vi "Write Read Loop with Config Speed Test eNames.vi"() -> (0 "error out":errorcluster)   [LabVIEW 2020]
panel:
  out "aValuesOut":dbl[][](array[numeric]) format="%.2f"
  in  "aNumValues":i32[](array[numeric])=[1, 1, 1, 1]
  in  "aWrites":i32[](array[ring])=[1, 1, 0, 0] items=["Read", "Write"]
  in  "aValuesIn":dbl[][](array[numeric])=[[2.34], [1.0]] format="%.2f"
  in  "aNames":string[](array[string])=["DAC0", "FIO1", "AIN0", "AIN1"]
  out "min ms":ext format="%.3g"
  out "max ms":ext format="%.3g"
  out "avg ms per iteration":ext format="%.3f"
  out "total ms":ext format="%.3g"
  out "Interval Array [ms] (Sorted Descending)":ext[](array[numeric]) format="%.3g"
  in  "Enable Interval Timing":bool=TRUE
  out "Interval Array [ms]":ext[](array[numeric]) format="%.3g"
  in  "# Iterations":i32=1000
  in  "Config Values":dbl[](array[numeric])=[10.0, 1.0] format="%.2f"
  in  "Config Names":string[](array[string])=["AIN_ALL_RANGE", "AIN_ALL_RESOLUTION_INDEX"]
  in  "Interval [ms]":i32
  out "Error String":string
  out "ConnectionType Out":i32
  out "DeviceType Out":i32
  in  "Identifier":string="LJM_idANY"
  in  "ConnectionType":string="LJM_ctANY"
  in  "DeviceType":string="LJM_dtANY"
  # "This modified version of a basic example adds code to do interval timing.  It does\nthe specified number of iterations and reports the average time per iteration.\n\nSet controls as desired then click arrow (upper-left of window) to run.  First the device is set to factory condition.  Then config values are written once before the loop.  Set Interval=0 to run as fast as possible.\n\nThis version uses 1 call to eNames to write and read."
  # "To remove an element, right-click on it, select\nData Operations => Remove Element.\n\nTo empty an array, right-click near the edge, select\nData Operations => Empty Array.\n\nOther useful operations:  From the Operate menu are \"Make Current\nValues Default\" and \"Reinitialize To Default\" (source only ... does\nnot work with exe)."
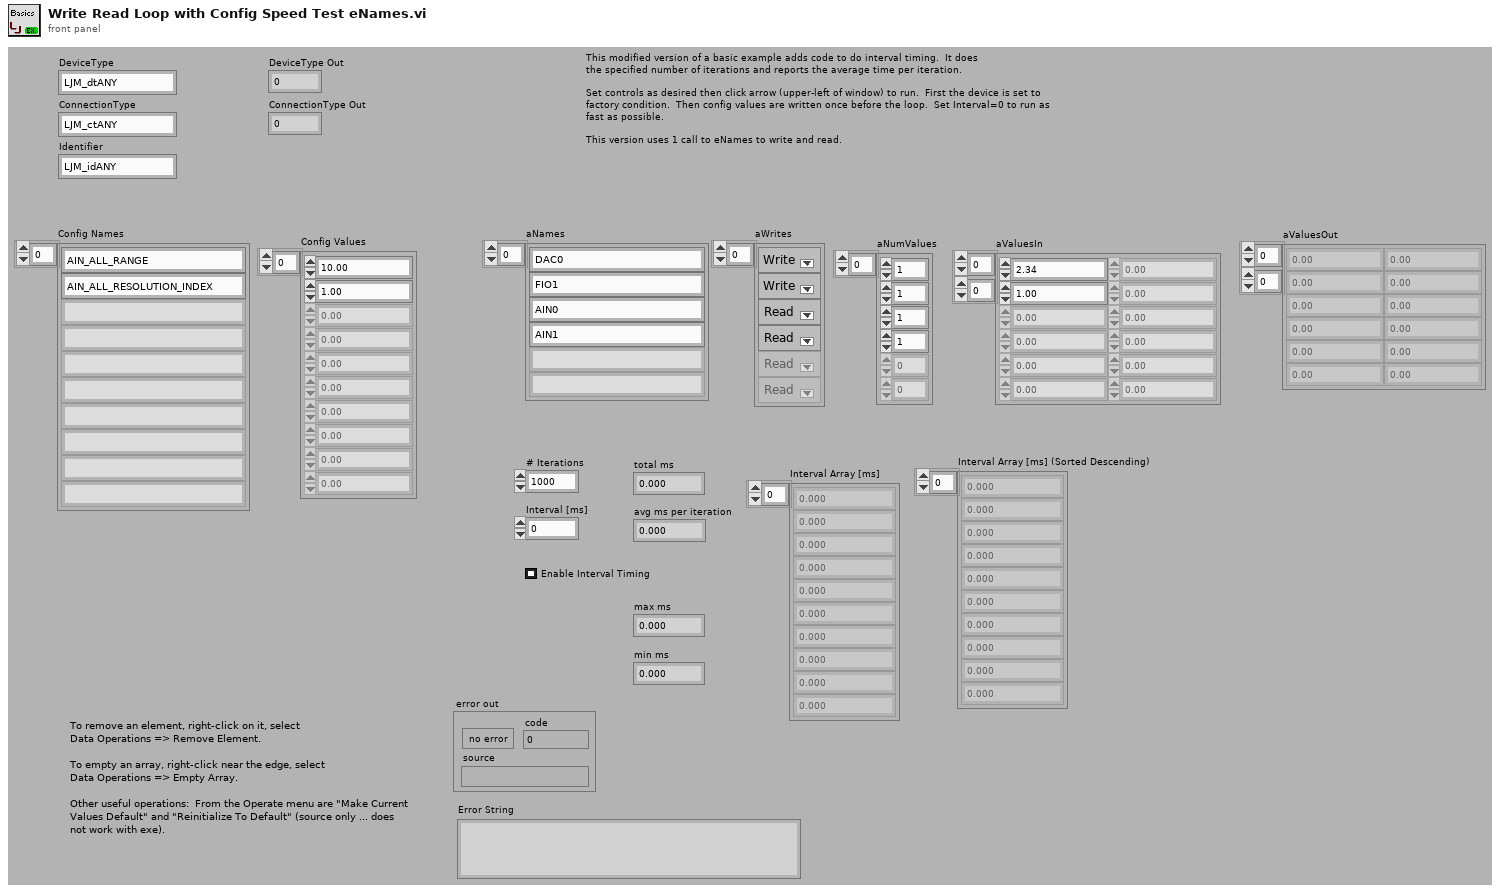
[diagram p1: front panel]
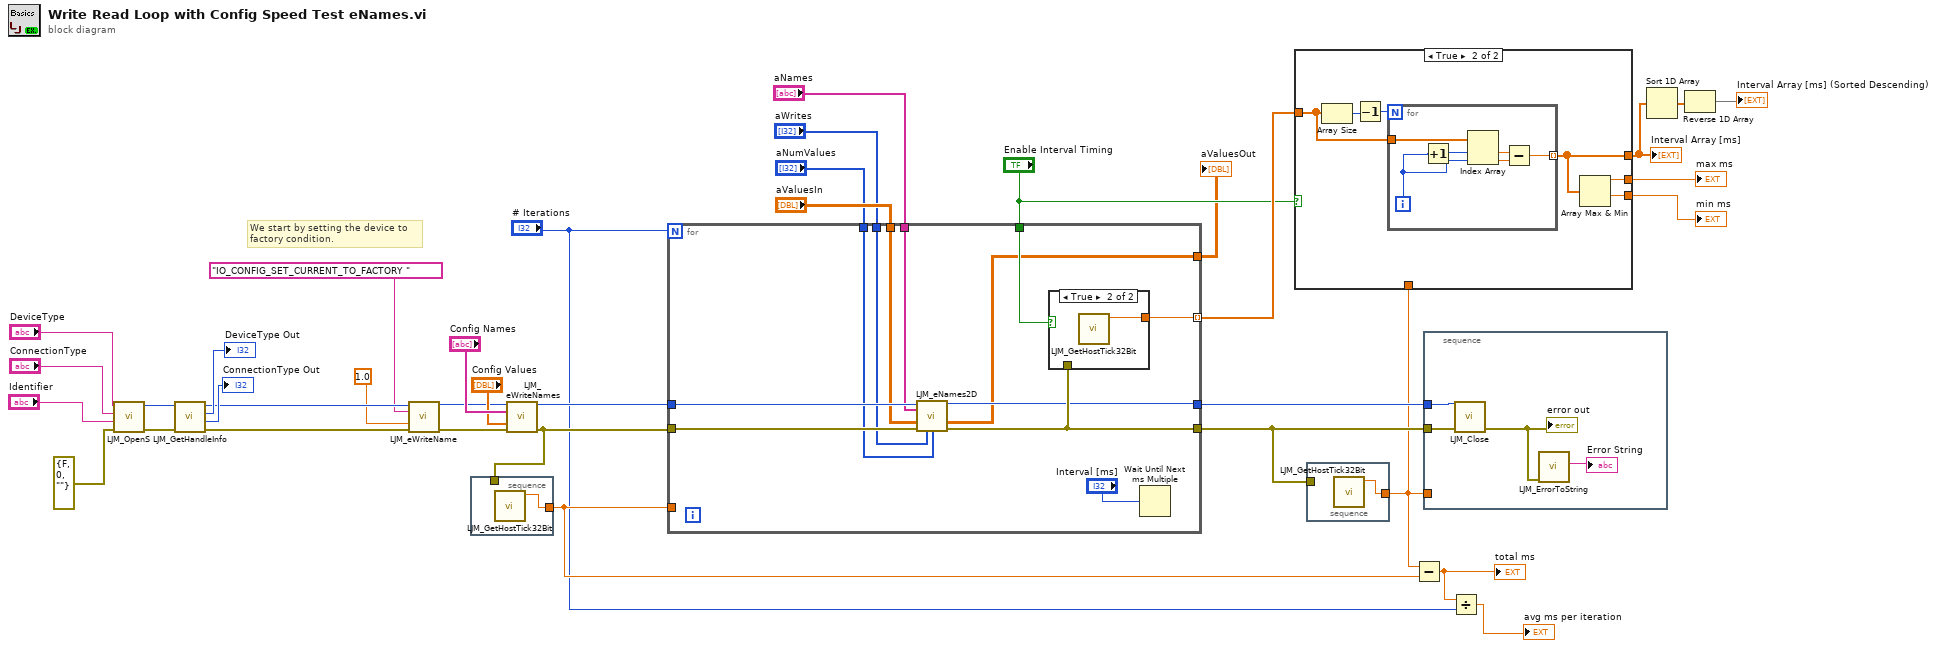
[diagram p0: block diagram]
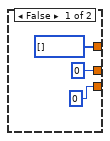
[diagram p2: hidden frame]
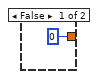
[diagram p3: hidden frame]
diagram:
  # "We start by setting the device to\nfactory condition."
  n1 = call "LJM_OpenS.vi"("error in"=errorcluster {"status"=FALSE, "code"=0, "source"=""} ("error in (no error)"), "Identifier"="Identifier", "ConnectionType"="ConnectionType", "DeviceType"="DeviceType") -> ("error out"=w36:errorcluster, "Handle"=w35:i32)  [unwired: 6 in]
  n2 = call "LJM_GetHandleInfo.vi"("error in"=w36, "Handle In"=w35) -> ("error out"=w7:errorcluster, "ConnectionType"=→"ConnectionType Out":i32, "DeviceType"=→"DeviceType Out":i32, "Handle Out"=w5:i32)  [unwired: 2 in, 4 out]
  n3 = call "LJM_eWriteName.vi"("Handle In"=w5, "Name"="IO_CONFIG_SET_CURRENT_TO_FACTORY ", "Value"=1.0, "error in"=w7) -> ("Handle Out"=w4:i32, "error out"=w6:errorcluster)  [unwired: 10 in]
  n4 = call "LJM_eWriteNames.vi"("Handle In"=w4, "aNames"="Config Names", "aValuesIn"="Config Values", "error in"=w6) -> ("Handle Out"=w29:i32, "error out"=w26:errorcluster)  [unwired: 9 in, 1 out]
  n5 = stacked-sequence {
    tunnel: [w38] -> w20
    tunnel: w26 -> [_]
    frame #0 {
      n6 = call "LJM_GetHostTick32Bit.vi"() -> ("Tick Ext [ms]"=w38:ext)  [unwired: 9 in, 2 out]
    }
  }
  n7 = for {
    N: "# Iterations" -> [_]
    tunnel: w26 -> [w45]
    tunnel: [w47] -> w22
    tunnel: w29 -> [w44]
    tunnel: [w46] -> w21
    tunnel: "Enable Interval Timing" -> [w49]
    tunnel: [w48] -> w18 mode=indexing
    tunnel: w20 -> [_]
    tunnel: "aNames" -> [w43]
    tunnel: "aValuesIn" -> [w42]
    tunnel: "aWrites" -> [w41]
    tunnel: "aNumValues" -> [w40]
    tunnel: [w39] -> w1
    n8 = call "LJM_eNames2D.vi"("Handle In"=w44, "aNames"=w43, "aValuesIn"=w42, "error in"=w45, "aWrites"=w41, "aNumValues"=w40) -> ("Handle Out"=w46:i32, "aValuesOut"=w39:dbl[][], "error out"=w47:errorcluster)  [unwired: 6 in, 1 out]
    n9 = case shown="True" w49 {
      tunnel: [u32 0 ("millisecond timer value") w52] -> w48
      tunnel: w47 -> [_ _]
      frame False {
      }
      frame True {
        n10 = call "LJM_GetHostTick32Bit.vi"() -> ("Tick Ext [ms]"=w52:ext)  [unwired: 9 in, 2 out]
      }
    }
    n11 = Wait Until Next ms Multiple(millisecond multiple="Interval [ms]") -> ()  [unwired: 1 out]
  }
  "aValuesOut" <- w1
  n12 = stacked-sequence {
    tunnel: [w53] -> w19
    tunnel: w22 -> [_]
    frame #0 {
      n13 = call "LJM_GetHostTick32Bit.vi"() -> ("Tick Ext [ms]"=w53:ext)  [unwired: 9 in, 2 out]
    }
  }
  n14 = case shown="True" "Enable Interval Timing" {
    tunnel: [u32[] [] w60] -> w13
    tunnel: [u32 0 w59] -> w15
    tunnel: [u32 0 w58] -> w14
    tunnel: w18 -> [_ w57]
    tunnel: w19 -> [_ _]
    frame False {
    }
    frame True {
      n15 = Array Size(array=w57) -> (size(s)=w62:i32)
      n16 = Decrement(x=w62) -> (x-1=w61:i32)
      n17 = for {
        N: w61 -> [_]
        tunnel: w57 -> [w68]
        tunnel: [w63] -> w60 mode=indexing
        i -> [w66]
        n18 = Increment(x=w66) -> (x+1=w67:i32)
        n19 = Index Array(array=w68, index #1=w67, index #2=w66) -> (element #1=w64:ext, element #2=w65:ext)
        n20 = Subtract(x=w64, y=w65) -> (x-y=w63:ext)
      }
      n21 = Array Max & Min(array=w60) -> (max value=w59:ext, min value=w58:ext)  [unwired: 2 out]
    }
  }
  "Interval Array [ms]" <- w13
  "max ms" <- w15
  "min ms" <- w14
  n22 = Subtract(x=w19, y=w20) -> (x-y=w24:ext)
  "total ms" <- w24
  n23 = stacked-sequence {
    tunnel: w22 -> [w72]
    tunnel: w19 -> [_]
    tunnel: w21 -> [w71]
    frame #0 {
      n24 = call "LJM_Close.vi"("error in"=w72, "Handle"=w71) -> ("error out"=w70:errorcluster)  [unwired: 9 in]
      "error out" <- w70
      n25 = call "LJM_ErrorToString.vi"("error in"=w70) -> ("String"=→"Error String":string)  [unwired: 10 in]
    }
  }
  n26 = Divide(x=w24, y="# Iterations") -> (x/y=→"avg ms per iteration":ext)
  n27 = Sort 1D Array(array=w13) -> (sorted array=w25:ext[])
  n28 = Reverse 1D Array(array=w25) -> (reversed array=→"Interval Array [ms] (Sorted Descending)":ext[])
